vi "draw_middle_lines.vi"(8 "error in (no error)":errorcluster, 10 "rotation angle":dbl[unit], 11 "Image in":refnum<class "Image.lvclass">) -> (0 "error out":errorcluster, 3 "Image out":refnum<class "Image.lvclass">)   [LabVIEW 2010, in "Image.lvclass"]
uses:
  Image.lvclass
  Image.lvclass/Image.ctl
  ErrorController/ErrorController/class_data.vi
  ErrorController/ErrorController/ErrorController.lvclass
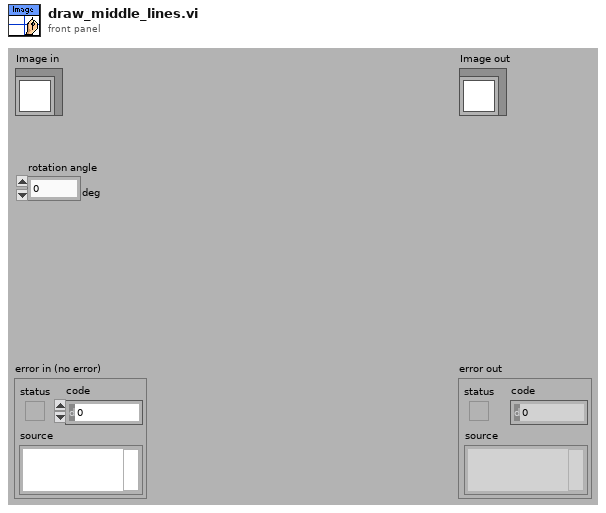
[diagram p1: front panel]
types:
  T1 = typedef "IMAQ Image.ctl" = refnum<image>
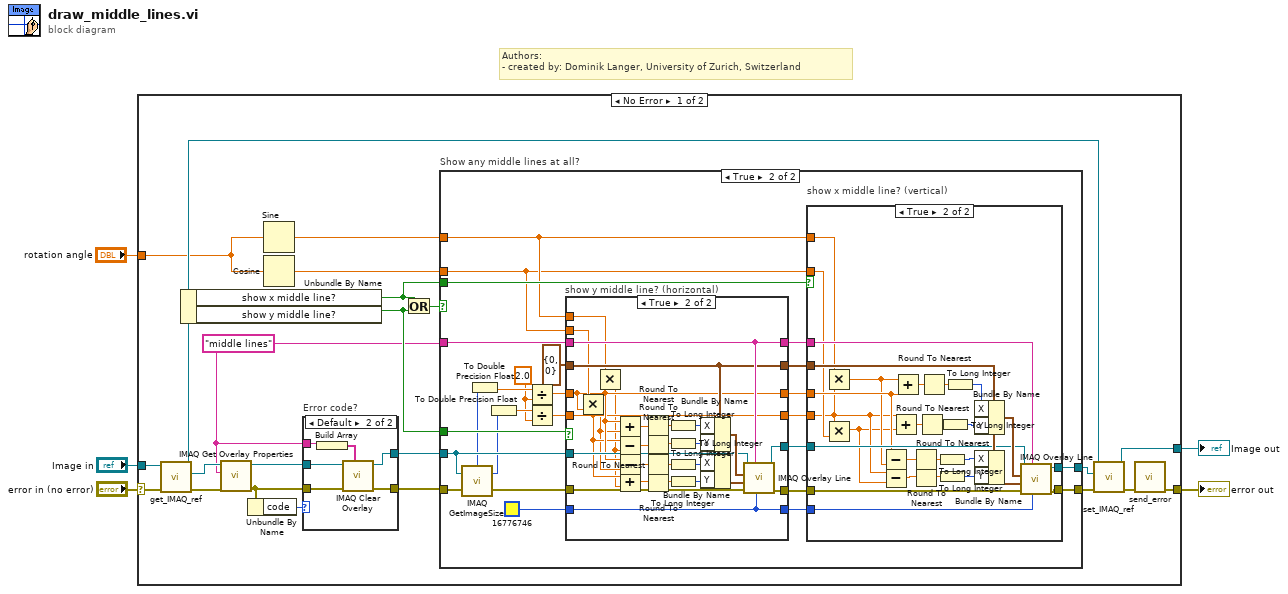
[diagram p0: block diagram]
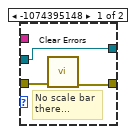
[diagram p2: hidden frame]
diagram:
  # "Authors: \n- created by: Dominik Langer, University of Zurich, Switzerland"
  n1 = case shown="No Error" "error in (no error)" {
    selector: "error in (no error)" -> [w24 w129]
    tunnel: [w6 w129] -> w4
    tunnel: [w21 w128] -> w2
    tunnel: "Image in" -> [w23 w128]
    tunnel: "rotation angle" -> [w10 _]
    frame No Error {
      w11 = "middle lines" ("String")
      n2 = call-dynamic "get_IMAQ_ref.vi"("error in (no error)"=w24, "Image.lvclass in"=w23) -> ("error out"=w18:errorcluster, "Image"=w17:T1, "Image.lvclass out"=w20:refnum<class "Image.lvclass">)  [unwired: 7 out]
      n3 = Unbundle By Name(w20) -> ("show x middle line?"=w25:bool, "show y middle line?"=w26:bool)
      n4 = call "IMAQ Get Overlay Properties"("error in (no error)"=w18, "Group"=w11, "Image"=w17) -> ("error out"=w15:errorcluster, "Image Out"=w13:T1)  [unwired: 5 out]
      n5 = Unbundle By Name(w15) -> ("code"=w16:i32)
      n6 = Sine(x=w10) -> (sin(x)=w9:dbl)
      n7 = Cosine(x=w10) -> (cos(x)=w8:dbl)
      n8 = case "Error code?" shown="Default" w16 {
        tunnel: [w29 w36] -> w14
        tunnel: [w28 w35] -> w12
        tunnel: w11 -> [_ w32]
        tunnel: w15 -> [w30 w33]
        tunnel: w13 -> [w28 w31]
        frame -1074395148 {
          # "No scale bar there..."
          n9 = call <vilib>:"Clear Errors.vi"("error in (no error)"=w30) -> ("error out"=w29:errorcluster)  [unwired: 6 out]
        }
        frame Default {
          n10 = Build Array(w32) -> (w34:string[])
          n11 = call "IMAQ Clear Overlay"("Groups"=w34, "error in (no error)"=w33, "Image"=w31) -> ("error out"=w36:errorcluster, "Image Out"=w35:T1)  [unwired: 7 out]
        }
      }
      n12 = Or(x=w25, y=w26) -> (x .or. y?=w27:bool)
      n13 = case "Show any middle lines at all?" shown="True" w27 {
        tunnel: w14 -> [w38 w54]
        tunnel: [w38 w53] -> w22
        tunnel: w26 -> [_ w64]
        tunnel: w25 -> [_ w59]
        tunnel: w12 -> [w37 w52]
        tunnel: w11 -> [_ w51]
        tunnel: [w37 w50] -> w19
        tunnel: w9 -> [_ w40]
        tunnel: w8 -> [_ w39]
        frame False {
        }
        frame True {
          w43 = 2.0 ("y")
          n14 = call "IMAQ GetImageSize"("Image"=w52, "error in (no error)"=w54) -> ("Y Resolution"=w46:i32, "X Resolution"=w47:i32, "error out"=w63:errorcluster)  [unwired: 2 out]
          n15 = To Double Precision Float(number=w47) -> (double precision float=w45:dbl)
          n16 = To Double Precision Float(number=w46) -> (double precision float=w44:dbl)
          n17 = Divide(x=w45, y=w43) -> (x/y=w42:dbl)
          n18 = Divide(x=w44, y=w43) -> (x/y=w41:dbl)
          n19 = case "show y middle line? (horizontal)" shown="True" w64 {
            tunnel: w63 -> [w100 w126]
            tunnel: cluster{"X":i32, "Y":i32} {"X"=0, "Y"=0} ("Start Point") -> [w97 w119]
            tunnel: w42 -> [w96 w104]
            tunnel: w51 -> [w99 w120]
            tunnel: w41 -> [w95 w103]
            tunnel: [w100 w123] -> w61
            tunnel: w52 -> [w98 w122]
            tunnel: [w98 w121] -> w60
            tunnel: [w99 w120] -> w58
            tunnel: [w97 w119] -> w57
            tunnel: [w96 w104] -> w56
            tunnel: [w95 w103] -> w55
            tunnel: [w94 w118] -> w49
            tunnel: u32 16776746 ("Color") -> [w94 w118]
            tunnel: w40 -> [_ w117]
            tunnel: w39 -> [_ w116]
            frame False {
            }
            frame True {
              n20 = Multiply(x=w116, y=w104) -> (x*y=w102:dbl)
              n21 = Multiply(x=w117, y=w104) -> (x*y=w101:dbl)
              n22 = Add(x=w104, y=w102) -> (x+y=w108:dbl)
              n23 = Subtract(x=w103, y=w101) -> (x-y=w107:dbl)
              n24 = Subtract(x=w104, y=w102) -> (x-y=w106:dbl)
              n25 = Add(x=w103, y=w101) -> (x+y=w105:dbl)
              n26 = Round To Nearest(number=w108) -> (nearest integer value=w127:dbl)
              n27 = Round To Nearest(number=w107) -> (nearest integer value=w115:dbl)
              n28 = Round To Nearest(number=w106) -> (nearest integer value=w114:dbl)
              n29 = Round To Nearest(number=w105) -> (nearest integer value=w113:dbl)
              n30 = To Long Integer(number=w127) -> (32bit integer=w112:i32)
              n31 = To Long Integer(number=w115) -> (32bit integer=w111:i32)
              n32 = To Long Integer(number=w114) -> (32bit integer=w110:i32)
              n33 = To Long Integer(number=w113) -> (32bit integer=w109:i32)
              n34 = Bundle By Name(cluster=w119, "X"=w112, "Y"=w111) -> (w125:cluster{"X":i32, "Y":i32})
              n35 = Bundle By Name(cluster=w119, "X"=w110, "Y"=w109) -> (w124:cluster{"X":i32, "Y":i32})
              n36 = call "IMAQ Overlay Line"("Color"=w118, "Group"=w120, "error in (no error)"=w126, "End Point"=w124, "Start Point"=w125, "Image"=w122) -> ("error out"=w123:errorcluster, "Image Out"=w121:T1)  [unwired: 4 out]
            }
          }
          n37 = case "show x middle line? (vertical)" shown="True" w59 {
            tunnel: w61 -> [w66 w92]
            tunnel: w57 -> [_ w89]
            tunnel: w58 -> [_ w88]
            tunnel: w60 -> [w65 w87]
            tunnel: [w66 w86] -> w53
            tunnel: w56 -> [_ w80]
            tunnel: w55 -> [_ w70]
            tunnel: [w65 w85] -> w50
            tunnel: w49 -> [_ w84]
            tunnel: w40 -> [_ w83]
            tunnel: w39 -> [_ w75]
            frame False {
            }
            frame True {
              n38 = Multiply(x=w83, y=w70) -> (x*y=w79:dbl)
              n39 = Multiply(x=w70, y=w75) -> (x*y=w69:dbl)
              n40 = Subtract(x=w80, y=w79) -> (x-y=w77:dbl)
              n41 = Subtract(x=w70, y=w69) -> (x-y=w71:dbl)
              n42 = Add(x=w70, y=w69) -> (x+y=w73:dbl)
              n43 = Add(x=w79, y=w80) -> (x+y=w82:dbl)
              n44 = Round To Nearest(number=w77) -> (nearest integer value=w78:dbl)
              n45 = Round To Nearest(number=w71) -> (nearest integer value=w72:dbl)
              n46 = Round To Nearest(number=w73) -> (nearest integer value=w74:dbl)
              n47 = Round To Nearest(number=w82) -> (nearest integer value=w93:dbl)
              n48 = To Long Integer(number=w78) -> (32bit integer=w76:i32)
              n49 = To Long Integer(number=w72) -> (32bit integer=w68:i32)
              n50 = To Long Integer(number=w74) -> (32bit integer=w67:i32)
              n51 = To Long Integer(number=w93) -> (32bit integer=w81:i32)
              n52 = Bundle By Name(cluster=w89, "X"=w81, "Y"=w67) -> (w91:cluster{"X":i32, "Y":i32})
              n53 = Bundle By Name(cluster=w89, "X"=w76, "Y"=w68) -> (w90:cluster{"X":i32, "Y":i32})
              n54 = call "IMAQ Overlay Line"("Color"=w84, "Group"=w88, "error in (no error)"=w92, "End Point"=w90, "Start Point"=w91, "Image"=w87) -> ("error out"=w86:errorcluster, "Image Out"=w85:T1)  [unwired: 4 out]
            }
          }
        }
      }
      n55 = call-dynamic "set_IMAQ_ref.vi"("error in (no error)"=w22, "Image"=w19, "Image.lvclass in"=w20) -> ("error out"=w7:errorcluster, "Image.lvclass out"=w21:refnum<class "Image.lvclass">)  [unwired: 7 out]
      n56 = call "send_error.vi"("error in (no error)"=w7) -> ("error out"=w6:errorcluster)  [unwired: 10 in]
    }
    frame Error {
    }
  }
  "error out" <- w4
  "Image out" <- w2
